vi "fail flag.vi"(7 "Command":enum16{"init", "read", "write"}(ring), 11 "Fail Index":bool[](array[boolean])) -> (3 "Fail Index Out":bool[](array[boolean]))   [LabVIEW 2016]
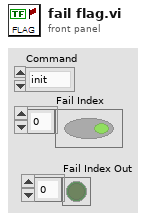
[diagram p1: front panel]
types:
  T1 = cluster{"Test Information":cluster{"date":string, "custom":string, "oper":string, "package":string, "pkg side":string, "solder":string, "brd side":string, "paste":string, "reflow":string}, "Sensor Set":cluster{"Accelerometer":cluster{"Sensitivity(mV/g)":dbl}, "Strain Guage":cluster{"Ch.":dbl[], "Gage factor":dbl[], "Resistance":dbl[], "Poisson ratio":dbl[]}}, "Resistor Set":cluster{"Criterion Level":dbl, "Res. Set":cluster{"Res. Ch":dbl, "Res. Active":bool, "Res Initial":dbl}[]}, "Test Stop Condition":cluster{"Test cycle":u16, "Fail number in a cycle":u16, "Fail factor":cluster{"Duration":u16, "Fail No.":u16}}, "Acceleration Condition ":cluster{"Shock duration pecent [%]":u16, "Filter cutoff freq":u32}, "Save":cluster{"Save Path":path, "File Name":string}}
  T2 = cluster{"Res. Ch":dbl, "Res. Active":bool, "Res Initial":dbl}[]
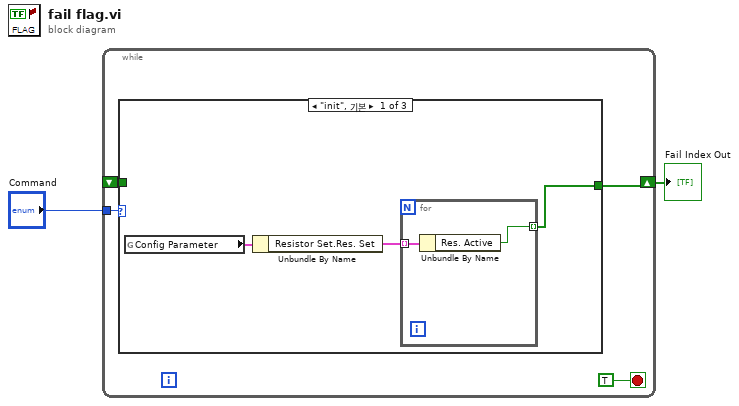
[diagram p0: block diagram]
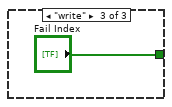
[diagram p3: hidden frame]
diagram:
  n1 = while {
    shift-right: [w4] -> w1
    shift-left: _ -> [w3]
    tunnel: "Command" -> [w5]
    stop <- TRUE stop-if-true
    n2 = case shown="\"init\", 기본" w5 {
      tunnel: [w7 w12 "Fail Index"] -> w4
      tunnel: w3 -> [_ w12 _]
      frame "init", Default {
        n3 = global read "글로벌_Config Parameter.vi" "Config Parameter"() -> (w9:T1)
        n4 = Unbundle By Name(w9) -> ("Resistor Set.Res. Set"=w8:T2)
        n5 = for {
          tunnel: w8 -> [w11] mode=indexing
          tunnel: [w10] -> w7 mode=indexing
          n6 = Unbundle By Name(w11) -> ("Res. Active"=w10:bool)
        }
      }
      frame "read" {
      }
      frame "write" {
      }
    }
  }
  "Fail Index Out" <- w1
